vi "Save Lockin Metadata.vi"(8 "error in (no error)":errorcluster, 11 "DAQmx Lockin Digitizer Driver in":refnum<class "DAQmx Lockin Digitizer Driver.lvclass">) -> (0 "error out":errorcluster, 3 "DAQmx Lockin Digitizer Driver out":refnum<class "DAQmx Lockin Digitizer Driver.lvclass">)   [LabVIEW 2024, in "DAQmx Lockin Digitizer Driver.lvclass"]
uses:
  DAQmx Lockin Digitizer Driver.lvclass
  Instruments/Pulse Driver/Pulse Driver.lvclass/Pulse Driver.ctl
  Instruments/Pulse Driver/Read tdms file.vi
  Instruments/Pulse Driver/Write tdms file.vi
  DAQmx Lockin Digitizer Driver.lvclass/DAQmx Lockin Digitizer Driver.ctl
  <resource>/objmgr/daqmx.rc
  DAQmx Lockin Driver/DAQmx Lockin Driver.lvclass
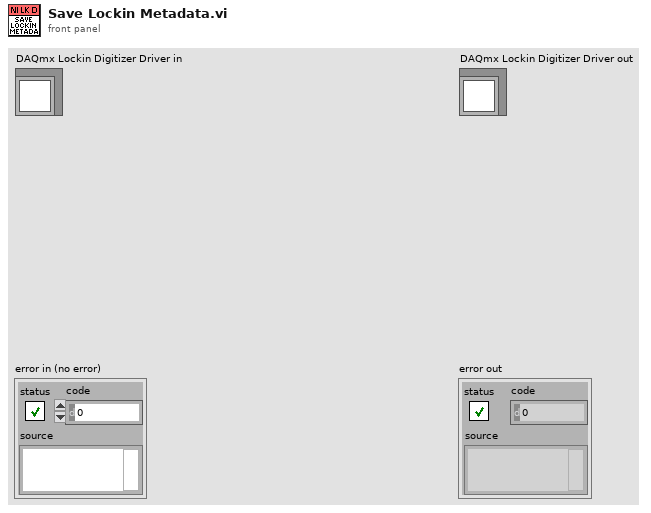
[diagram p1: front panel]
types:
  T1 = typedef "Lockin Digitizer Configuration.ctl" = cluster{"Post-trigger delay":dbl, "Post-trigger duration":dbl, "Rate":dbl, "Ranges":dbl[], "Re-name channels":string[], "Active channels":string, "External\nclock":bool, "Frequencies":dbl[], "Monitor time\nconstant":dbl, "Output \namplitudes":dbl[], "Input\nchannles":string[], "Sync":bool, "Lock-in input channel phases":dbl[]}
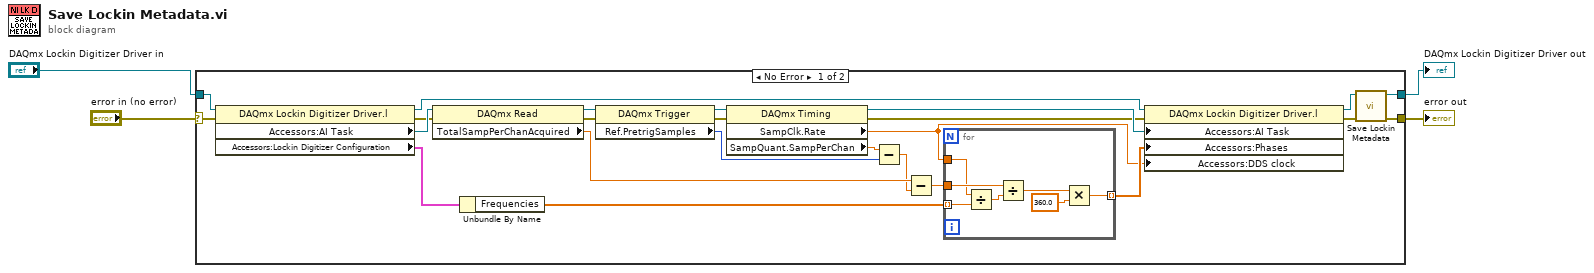
[diagram p0: block diagram]
diagram:
  n1 = case shown="No Error" "error in (no error)" {
    selector: "error in (no error)" -> [w28 w37]
    tunnel: [w7 w37] -> w3
    tunnel: [w9 w36] -> w1
    tunnel: "DAQmx Lockin Digitizer Driver in" -> [w11 w36]
    frame No Error {
      n2 = property class="DAQmx Lockin Digitizer Driver.l"(reference=w11, error in=w28) -> (reference out=w12:refnum<class "DAQmx Lockin Digitizer Driver.lvclass">, error out=w24:errorcluster, "Accessors:AI Task"=w25:refnum<k21>, "Accessors:Lockin Digitizer Configuration"=w27:T1)
      n3 = property class="DAQmx Read"(reference=w25, error in=w24) -> (reference out=w18:refnum<k21>, error out=w17:errorcluster, "TotalSampPerChanAcquired"=w23:dbl)
      n4 = Unbundle By Name(w27) -> ("Frequencies"=w26:dbl[])
      n5 = property class="DAQmx Trigger"(reference=w18, error in=w17) -> (reference out=w16:refnum<k21>, error out=w15:errorcluster, "Ref.PretrigSamples"=w22:u32)
      n6 = property class="DAQmx Timing"(reference=w16, error in=w15) -> (reference out=w13:refnum<k21>, error out=w5:errorcluster, "SampClk.Rate"=w6:dbl, "SampQuant.SampPerChan"=w19:dbl)
      n7 = Subtract(x=w19, y=w22) -> (x-y=w21:dbl)
      n8 = Subtract(x=w23, y=w21) -> (x-y=w20:dbl)
      n9 = for {
        tunnel: w26 -> [w35] mode=indexing
        tunnel: w6 -> [w30]
        tunnel: w20 -> [w34]
        tunnel: [w29] -> w10 mode=indexing
        n10 = Divide(x=w30, y=w35) -> (x/y=w33:dbl)
        n11 = Divide(x=w34, y=w33) -> (x/y=w32:dbl)
        n12 = Multiply(x=w32, y=360.0) -> (x*y=w29:dbl)
      }
      n13 = property class="DAQmx Lockin Digitizer Driver.l"(reference=w12, error in=w5, "Accessors:AI Task"=w13, "Accessors:Phases"=w10, "Accessors:DDS clock"=w6) -> (reference out=w14:refnum<class "DAQmx Lockin Digitizer Driver.lvclass">, error out=w8:errorcluster)
      n14 = call-parent "Save Lockin Metadata.vi"("error in (no error)"=w8, "Lockin Digitizer Driver in"=w14) -> ("error out"=w7:errorcluster, "Lockin Digitizer Driver out"=w9:refnum<class "DAQmx Lockin Digitizer Driver.lvclass">)  [unwired: 8 in]
    }
    frame Error {
    }
  }
  "error out" <- w3
  "DAQmx Lockin Digitizer Driver out" <- w1
